vi "GetFileNames.vi"(7 "LabVIEW Web Service Request":refnum<class "Web Request.lvclass">) -> ()   [LabVIEW 2019]
uses:
  <vilib>/wsapi/Web Request.lvclass
  IndoorData_class/IndoorData.lvclass
panel:
  # "Use the Web Service Request input terminal to call the VIs on the Web Services palette. Do not remove it from the connector pane unless you don't need access to the palette."
  # "Each additional control wired to the connector pane will be available as an input in the URL. To include an indicator in terminal-mode output (the default setting), it must also be wired to the connector pane."
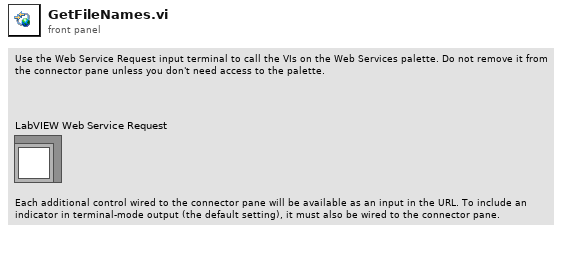
[diagram p1: front panel]
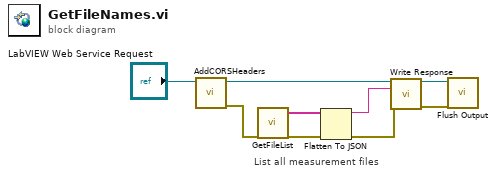
[diagram p0: block diagram]
diagram:
  # "List all measurement files"
  n1 = call "AddCORSHeaders.vi"("LabVIEW Web Service Request"="LabVIEW Web Service Request") -> ("error out"=w7:errorcluster, "LabVIEW Web Service Request out"=w6:refnum<class "Web Request.lvclass">)  [unwired: 9 in]
  n2 = call "GetFileList.vi"("error in (no error)"=w7) -> ("filenames"=w4:string[], "error out"=w5:errorcluster)  [unwired: 17 in]
  n3 = Flatten To JSON(anything=w4, error in (no error)=w5) -> (JSON string=w3:string, 11:w2:errorcluster)  [unwired: 1 in]
  n4 = call <vilib>:"Write Response.vi"("LabVIEW Web Service Request"=w6, "response string"=w3, "error in (no error)"=w2) -> ("LabVIEW Web Service Request out"=w9:refnum<class "Web Request.lvclass">, "error out"=w8:errorcluster)  [unwired: 11 in]
  n5 = call <vilib>:"Flush Output.vi"("LabVIEW Web Service Request"=w9, "error in (no error)"=w8) -> ()  [unwired: 12 in, 2 out]
